vi "ReplaceInMatriceScaling.vi"(8 "Input Scaling":i32=4, 11 "Input Array":dbl[](array[numeric])) -> (0 "Output Array":dbl[][](array[numeric]))   [LabVIEW 2018]
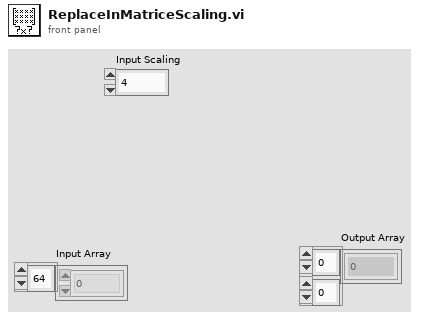
[diagram p1: front panel]
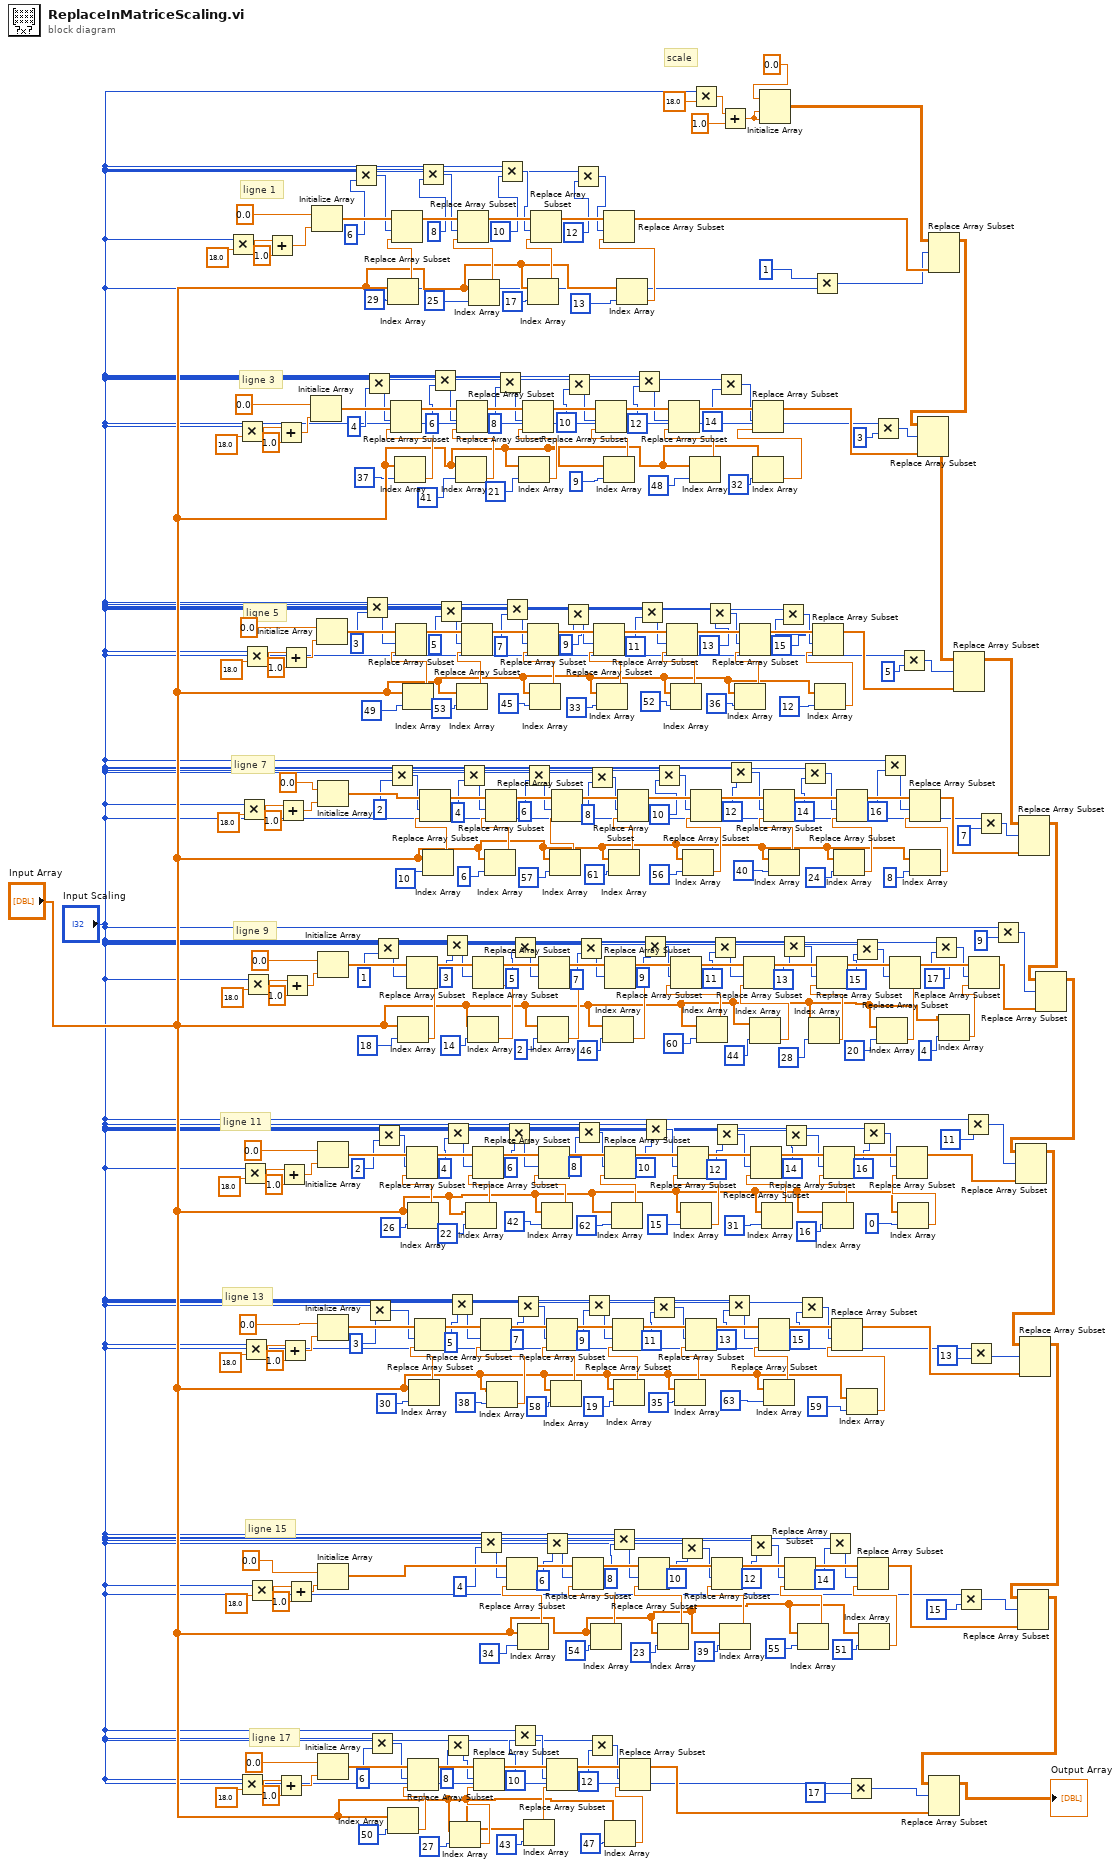
[diagram p0: block diagram]
diagram:
  # "scale"
  # "ligne 17"
  # "ligne 15"
  # "ligne 13"
  # "ligne 11"
  # "ligne 9"
  # "ligne 7"
  # "ligne 5"
  # "ligne 3"
  # "ligne 1"
  n1 = Multiply(x="Input Scaling", y=18.0) -> (x*y=w232:dbl)
  n2 = Multiply(x="Input Scaling", y=18.0) -> (x*y=w228:dbl)
  n3 = Multiply(x="Input Scaling", y=18.0) -> (x*y=w200:dbl)
  n4 = Multiply(x="Input Scaling", y=18.0) -> (x*y=w220:dbl)
  n5 = Multiply(x="Input Scaling", y=18.0) -> (x*y=w212:dbl)
  n6 = Multiply(x="Input Scaling", y=18.0) -> (x*y=w208:dbl)
  n7 = Multiply(x="Input Scaling", y=18.0) -> (x*y=w224:dbl)
  n8 = Multiply(x="Input Scaling", y=18.0) -> (x*y=w216:dbl)
  n9 = Multiply(x="Input Scaling", y=18.0) -> (x*y=w204:dbl)
  n10 = Add(x=w232, y=1.0) -> (x+y=w230:dbl)
  n11 = Add(x=w228, y=1.0) -> (x+y=w226:dbl)
  n12 = Add(x=w200, y=1.0) -> (x+y=w198:dbl)
  n13 = Add(x=w220, y=1.0) -> (x+y=w218:dbl)
  n14 = Add(x=w212, y=1.0) -> (x+y=w210:dbl)
  n15 = Add(x=w208, y=1.0) -> (x+y=w206:dbl)
  n16 = Add(x=w224, y=1.0) -> (x+y=w222:dbl)
  n17 = Add(x=w216, y=1.0) -> (x+y=w214:dbl)
  n18 = Add(x=w204, y=1.0) -> (x+y=w202:dbl)
  n19 = Initialize Array(0.0 ("element"), w226) -> (w372:dbl[])
  n20 = Initialize Array(0.0 ("element"), w230) -> (w382:dbl[])
  n21 = Initialize Array(0.0 ("element"), w222) -> (w365:dbl[])
  n22 = Initialize Array(0.0 ("element"), w218) -> (w356:dbl[])
  n23 = Initialize Array(0.0 ("element"), w214) -> (w347:dbl[])
  n24 = Initialize Array(0.0 ("element"), w210) -> (w338:dbl[])
  n25 = Initialize Array(0.0 ("element"), w206) -> (w330:dbl[])
  n26 = Initialize Array(0.0 ("element"), w202) -> (w322:dbl[])
  n27 = Initialize Array(0.0 ("element"), w198) -> (w320:dbl[])
  n28 = Multiply(x="Input Scaling", y=6 ("index")) -> (x*y=w195:i32)
  n29 = Multiply(x="Input Scaling", y=3 ("index")) -> (x*y=w176:i32)
  n30 = Multiply(x="Input Scaling", y=4 ("index")) -> (x*y=w187:i32)
  n31 = Multiply(x="Input Scaling", y=3 ("index")) -> (x*y=w112:i32)
  n32 = Multiply(x="Input Scaling", y=6 ("index")) -> (x*y=w86:i32)
  n33 = Multiply(x="Input Scaling", y=1 ("index")) -> (x*y=w146:i32)
  n34 = Multiply(x="Input Scaling", y=2 ("index")) -> (x*y=w128:i32)
  n35 = Multiply(x="Input Scaling", y=2 ("index")) -> (x*y=w162:i32)
  n36 = Index Array(array="Input Array", index=29) -> (element=w305:dbl)
  n37 = Index Array(array="Input Array", index=50) -> (element=w259:dbl)
  n38 = Replace Array Subset(array=w382, new element=w305, index=w195) -> (w381:dbl[])
  n39 = Index Array(array="Input Array", index=37) -> (element=w304:dbl)
  n40 = Replace Array Subset(array=w372, new element=w304, index=w187) -> (w373:dbl[])
  n41 = Index Array(array="Input Array", index=18) -> (element=w316:dbl)
  n42 = Index Array(array="Input Array", index=49) -> (element=w298:dbl)
  n43 = Replace Array Subset(array=w365, new element=w298, index=w176) -> (w366:dbl[])
  n44 = Replace Array Subset(array=w347, new element=w316, index=w146) -> (w346:dbl[])
  n45 = Index Array(array="Input Array", index=26) -> (element=w276:dbl)
  n46 = Replace Array Subset(array=w338, new element=w276, index=w128) -> (w339:dbl[])
  n47 = Replace Array Subset(array=w320, new element=w259, index=w86) -> (w319:dbl[])
  n48 = Index Array(array="Input Array", index=30) -> (element=w275:dbl)
  n49 = Replace Array Subset(array=w330, new element=w275, index=w112) -> (w331:dbl[])
  n50 = Multiply(x="Input Scaling", y=8 ("index")) -> (x*y=w190:i32)
  n51 = Index Array(array="Input Array", index=10) -> (element=w291:dbl)
  n52 = Replace Array Subset(array=w356, new element=w291, index=w162) -> (w357:dbl[])
  n53 = Multiply(x="Input Scaling", y=6 ("index")) -> (x*y=w185:i32)
  n54 = Multiply(x="Input Scaling", y=5 ("index")) -> (x*y=w174:i32)
  n55 = Multiply(x="Input Scaling", y=3 ("index")) -> (x*y=w144:i32)
  n56 = Multiply(x="Input Scaling", y=4 ("index")) -> (x*y=w126:i32)
  n57 = Multiply(x="Input Scaling", y=8 ("index")) -> (x*y=w84:i32)
  n58 = Multiply(x="Input Scaling", y=5 ("index")) -> (x*y=w110:i32)
  n59 = Index Array(array="Input Array", index=27) -> (element=w260:dbl)
  n60 = Index Array(array="Input Array", index=41) -> (element=w303:dbl)
  n61 = Replace Array Subset(array=w373, new element=w303, index=w185) -> (w377:dbl[])
  n62 = Index Array(array="Input Array", index=53) -> (element=w297:dbl)
  n63 = Multiply(x="Input Scaling", y=4 ("index")) -> (x*y=w160:i32)
  n64 = Replace Array Subset(array=w366, new element=w297, index=w174) -> (w370:dbl[])
  n65 = Index Array(array="Input Array", index=22) -> (element=w277:dbl)
  n66 = Index Array(array="Input Array", index=14) -> (element=w315:dbl)
  n67 = Index Array(array="Input Array", index=25) -> (element=w306:dbl)
  n68 = Replace Array Subset(array=w381, new element=w306, index=w190) -> (w380:dbl[])
  n69 = Replace Array Subset(array=w346, new element=w315, index=w144) -> (w349:dbl[])
  n70 = Replace Array Subset(array=w339, new element=w277, index=w126) -> (w340:dbl[])
  n71 = Replace Array Subset(array=w319, new element=w260, index=w84) -> (w318:dbl[])
  n72 = Multiply(x="Input Scaling", y=4 ("index")) -> (x*y=w98:i32)
  n73 = Index Array(array="Input Array", index=6) -> (element=w290:dbl)
  n74 = Replace Array Subset(array=w357, new element=w290, index=w160) -> (w358:dbl[])
  n75 = Index Array(array="Input Array", index=38) -> (element=w274:dbl)
  n76 = Replace Array Subset(array=w331, new element=w274, index=w110) -> (w335:dbl[])
  n77 = Multiply(x="Input Scaling", y=8 ("index")) -> (x*y=w184:i32)
  n78 = Multiply(x="Input Scaling", y=10 ("index")) -> (x*y=w191:i32)
  n79 = Multiply(x="Input Scaling", y=7 ("index")) -> (x*y=w172:i32)
  n80 = Multiply(x="Input Scaling", y=6 ("index")) -> (x*y=w124:i32)
  n81 = Multiply(x="Input Scaling", y=5 ("index")) -> (x*y=w142:i32)
  n82 = Multiply(x="Input Scaling", y=10 ("index")) -> (x*y=w82:i32)
  n83 = Multiply(x="Input Scaling", y=7 ("index")) -> (x*y=w108:i32)
  n84 = Index Array(array="Input Array", index=34) -> (element=w263:dbl)
  n85 = Replace Array Subset(array=w322, new element=w263, index=w98) -> (w323:dbl[])
  n86 = Index Array(array="Input Array", index=21) -> (element=w299:dbl)
  n87 = Replace Array Subset(array=w377, new element=w299, index=w184) -> (w376:dbl[])
  n88 = Multiply(x="Input Scaling", y=6 ("index")) -> (x*y=w157:i32)
  n89 = Index Array(array="Input Array", index=43) -> (element=w261:dbl)
  n90 = Index Array(array="Input Array", index=17) -> (element=w307:dbl)
  n91 = Index Array(array="Input Array", index=45) -> (element=w296:dbl)
  n92 = Replace Array Subset(array=w370, new element=w296, index=w172) -> (w369:dbl[])
  n93 = Replace Array Subset(array=w380, new element=w307, index=w191) -> (w379:dbl[])
  n94 = Index Array(array="Input Array", index=2) -> (element=w314:dbl)
  n95 = Replace Array Subset(array=w349, new element=w314, index=w142) -> (w353:dbl[])
  n96 = Index Array(array="Input Array", index=42) -> (element=w278:dbl)
  n97 = Replace Array Subset(array=w340, new element=w278, index=w124) -> (w344:dbl[])
  n98 = Multiply(x="Input Scaling", y=6 ("index")) -> (x*y=w96:i32)
  n99 = Replace Array Subset(array=w318, new element=w261, index=w82) -> (w317:dbl[])
  n100 = Index Array(array="Input Array", index=57) -> (element=w289:dbl)
  n101 = Index Array(array="Input Array", index=58) -> (element=w273:dbl)
  n102 = Replace Array Subset(array=w335, new element=w273, index=w108) -> (w334:dbl[])
  n103 = Replace Array Subset(array=w358, new element=w289, index=w157) -> (w362:dbl[])
  n104 = Multiply(x="Input Scaling", y=9 ("index")) -> (x*y=w170:i32)
  n105 = Multiply(x="Input Scaling", y=10 ("index")) -> (x*y=w182:i32)
  n106 = Multiply(x="Input Scaling", y=12 ("index")) -> (x*y=w194:i32)
  n107 = Multiply(x="Input Scaling", y=8 ("index")) -> (x*y=w122:i32)
  n108 = Multiply(x="Input Scaling", y=7 ("index")) -> (x*y=w140:i32)
  n109 = Multiply(x="Input Scaling", y=9 ("index")) -> (x*y=w106:i32)
  n110 = Multiply(x="Input Scaling", y=8 ("index")) -> (x*y=w156:i32)
  n111 = Multiply(x="Input Scaling", y=12 ("index")) -> (x*y=w80:i32)
  n112 = Index Array(array="Input Array", index=54) -> (element=w264:dbl)
  n113 = Replace Array Subset(array=w323, new element=w264, index=w96) -> (w327:dbl[])
  n114 = Index Array(array="Input Array", index=33) -> (element=w295:dbl)
  n115 = Replace Array Subset(array=w369, new element=w295, index=w170) -> (w368:dbl[])
  n116 = Index Array(array="Input Array", index=46) -> (element=w313:dbl)
  n117 = Index Array(array="Input Array", index=9) -> (element=w300:dbl)
  n118 = Replace Array Subset(array=w376, new element=w300, index=w182) -> (w375:dbl[])
  n119 = Replace Array Subset(array=w353, new element=w313, index=w140) -> (w352:dbl[])
  n120 = Index Array(array="Input Array", index=47) -> (element=w262:dbl)
  n121 = Index Array(array="Input Array", index=61) -> (element=w288:dbl)
  n122 = Multiply(x="Input Scaling", y=8 ("index")) -> (x*y=w94:i32)
  n123 = Index Array(array="Input Array", index=62) -> (element=w279:dbl)
  n124 = Replace Array Subset(array=w344, new element=w279, index=w122) -> (w343:dbl[])
  n125 = Index Array(array="Input Array", index=19) -> (element=w272:dbl)
  n126 = Replace Array Subset(array=w334, new element=w272, index=w106) -> (w333:dbl[])
  n127 = Index Array(array="Input Array", index=13) -> (element=w308:dbl)
  n128 = Replace Array Subset(array=w379, new element=w308, index=w194) -> (w257:dbl[])
  n129 = Replace Array Subset(array=w362, new element=w288, index=w156) -> (w361:dbl[])
  n130 = Replace Array Subset(array=w317, new element=w262, index=w80) -> (w242:dbl[])
  n131 = Multiply(x="Input Scaling", y=12 ("index")) -> (x*y=w180:i32)
  n132 = Multiply(x="Input Scaling", y=11 ("index")) -> (x*y=w168:i32)
  n133 = Multiply(x="Input Scaling", y=9 ("index")) -> (x*y=w138:i32)
  n134 = Multiply(x="Input Scaling", y=10 ("index")) -> (x*y=w120:i32)
  n135 = Multiply(x="Input Scaling", y=11 ("index")) -> (x*y=w104:i32)
  n136 = Multiply(x="Input Scaling", y=10 ("index")) -> (x*y=w154:i32)
  n137 = Index Array(array="Input Array", index=23) -> (element=w265:dbl)
  n138 = Replace Array Subset(array=w327, new element=w265, index=w94) -> (w326:dbl[])
  n139 = Index Array(array="Input Array", index=52) -> (element=w294:dbl)
  n140 = Replace Array Subset(array=w368, new element=w294, index=w168) -> (w367:dbl[])
  n141 = Index Array(array="Input Array", index=35) -> (element=w271:dbl)
  n142 = Multiply(x="Input Scaling", y=10 ("index")) -> (x*y=w92:i32)
  n143 = Index Array(array="Input Array", index=15) -> (element=w280:dbl)
  n144 = Replace Array Subset(array=w343, new element=w280, index=w120) -> (w342:dbl[])
  n145 = Index Array(array="Input Array", index=56) -> (element=w287:dbl)
  n146 = Replace Array Subset(array=w333, new element=w271, index=w104) -> (w332:dbl[])
  n147 = Index Array(array="Input Array", index=48) -> (element=w301:dbl)
  n148 = Replace Array Subset(array=w375, new element=w301, index=w180) -> (w374:dbl[])
  n149 = Multiply(x="Input Scaling", y=18.0) -> (x*y=w235:dbl)
  n150 = Replace Array Subset(array=w361, new element=w287, index=w154) -> (w360:dbl[])
  n151 = Index Array(array="Input Array", index=60) -> (element=w312:dbl)
  n152 = Replace Array Subset(array=w352, new element=w312, index=w138) -> (w351:dbl[])
  n153 = Multiply(x="Input Scaling", y=13 ("index")) -> (x*y=w166:i32)
  n154 = Multiply(x="Input Scaling", y=11 ("index")) -> (x*y=w136:i32)
  n155 = Multiply(x="Input Scaling", y=12 ("index")) -> (x*y=w118:i32)
  n156 = Multiply(x="Input Scaling", y=14 ("index")) -> (x*y=w178:i32)
  n157 = Add(x=w235, y=1.0) -> (x+y=w236:dbl)
  n158 = Index Array(array="Input Array", index=39) -> (element=w266:dbl)
  n159 = Replace Array Subset(array=w326, new element=w266, index=w92) -> (w325:dbl[])
  n160 = Multiply(x="Input Scaling", y=13 ("index")) -> (x*y=w102:i32)
  n161 = Multiply(x="Input Scaling", y=12 ("index")) -> (x*y=w152:i32)
  n162 = Index Array(array="Input Array", index=36) -> (element=w293:dbl)
  n163 = Replace Array Subset(array=w367, new element=w293, index=w166) -> (w364:dbl[])
  n164 = Multiply(x="Input Scaling", y=12 ("index")) -> (x*y=w90:i32)
  n165 = Index Array(array="Input Array", index=44) -> (element=w311:dbl)
  n166 = Replace Array Subset(array=w351, new element=w311, index=w136) -> (w350:dbl[])
  n167 = Index Array(array="Input Array", index=32) -> (element=w302:dbl)
  n168 = Replace Array Subset(array=w374, new element=w302, index=w178) -> (w248:dbl[])
  n169 = Initialize Array(0.0, w236, w236) -> (w258:dbl[][])
  n170 = Index Array(array="Input Array", index=31) -> (element=w281:dbl)
  n171 = Replace Array Subset(array=w342, new element=w281, index=w118) -> (w341:dbl[])
  n172 = Index Array(array="Input Array", index=63) -> (element=w270:dbl)
  n173 = Replace Array Subset(array=w332, new element=w270, index=w102) -> (w329:dbl[])
  n174 = Index Array(array="Input Array", index=40) -> (element=w286:dbl)
  n175 = Replace Array Subset(array=w360, new element=w286, index=w152) -> (w359:dbl[])
  n176 = Multiply(x="Input Scaling", y=15 ("index")) -> (x*y=w164:i32)
  n177 = Multiply(x="Input Scaling", y=13 ("index")) -> (x*y=w134:i32)
  n178 = Multiply(x="Input Scaling", y=14 ("index")) -> (x*y=w116:i32)
  n179 = Multiply(x="Input Scaling", y=15 ("index")) -> (x*y=w100:i32)
  n180 = Index Array(array="Input Array", index=55) -> (element=w267:dbl)
  n181 = Replace Array Subset(array=w325, new element=w267, index=w90) -> (w324:dbl[])
  n182 = Multiply(x="Input Scaling", y=14 ("index")) -> (x*y=w150:i32)
  n183 = Index Array(array="Input Array", index=28) -> (element=w310:dbl)
  n184 = Multiply(x=1 ("index (row)"), y="Input Scaling") -> (x*y=w77:i32)
  n185 = Index Array(array="Input Array", index=12) -> (element=w292:dbl)
  n186 = Replace Array Subset(array=w364, new element=w292, index=w164) -> (w247:dbl[])
  n187 = Replace Array Subset(array=w350, new element=w310, index=w134) -> (w348:dbl[])
  n188 = Index Array(array="Input Array", index=16) -> (element=w282:dbl)
  n189 = Replace Array Subset(array=w341, new element=w282, index=w116) -> (w337:dbl[])
  n190 = Multiply(x="Input Scaling", y=14 ("index")) -> (x*y=w88:i32)
  n191 = Index Array(array="Input Array", index=24) -> (element=w285:dbl)
  n192 = Replace Array Subset(array=w359, new element=w285, index=w150) -> (w355:dbl[])
  n193 = Multiply(x="Input Scaling", y=17 ("index (row)")) -> (x*y=w62:i32)
  n194 = Index Array(array="Input Array", index=59) -> (element=w269:dbl)
  n195 = Replace Array Subset(array=w329, new element=w269, index=w100) -> (w244:dbl[])
  n196 = Multiply(x="Input Scaling", y=15 ("index")) -> (x*y=w132:i32)
  n197 = Multiply(x="Input Scaling", y=16 ("index")) -> (x*y=w114:i32)
  n198 = Index Array(array="Input Array", index=51) -> (element=w268:dbl)
  n199 = Replace Array Subset(array=w324, new element=w268, index=w88) -> (w243:dbl[])
  n200 = Multiply(x="Input Scaling", y=3 ("index (row)")) -> (x*y=w76:i32)
  n201 = Index Array(array="Input Array", index=20) -> (element=w309:dbl)
  n202 = Multiply(x="Input Scaling", y=16 ("index")) -> (x*y=w148:i32)
  n203 = Replace Array Subset(array=w348, new element=w309, index=w132) -> (w240:dbl[])
  n204 = Index Array(array="Input Array", index=0) -> (element=w283:dbl)
  n205 = Replace Array Subset(array=w337, new element=w283, index=w114) -> (w245:dbl[])
  n206 = Multiply(x="Input Scaling", y=5 ("index (row)")) -> (x*y=w73:i32)
  n207 = Index Array(array="Input Array", index=8) -> (element=w284:dbl)
  n208 = Replace Array Subset(array=w355, new element=w284, index=w148) -> (w246:dbl[])
  n209 = Replace Array Subset(array=w258, new element=w257, index (row)=w77) -> (w256:dbl[][])  [unwired: 1 in]
  n210 = Replace Array Subset(array=w256, new element=w248, index (row)=w76) -> (w255:dbl[][])  [unwired: 1 in]
  n211 = Multiply(x="Input Scaling", y=17 ("index")) -> (x*y=w130:i32)
  n212 = Index Array(array="Input Array", index=4) -> (element=w238:dbl)
  n213 = Replace Array Subset(array=w255, new element=w247, index (row)=w73) -> (w254:dbl[][])  [unwired: 1 in]
  n214 = Multiply(x="Input Scaling", y=15 ("index (row)")) -> (x*y=w63:i32)
  n215 = Multiply(x="Input Scaling", y=11 ("index (row)")) -> (x*y=w67:i32)
  n216 = Multiply(x="Input Scaling", y=13 ("index (row)")) -> (x*y=w66:i32)
  n217 = Replace Array Subset(array=w240, new element=w238, index=w130) -> (w239:dbl[])
  n218 = Multiply(x="Input Scaling", y=7 ("index (row)")) -> (x*y=w71:i32)
  n219 = Multiply(x="Input Scaling", y=9 ("index (row)")) -> (x*y=w70:i32)
  n220 = Replace Array Subset(array=w254, new element=w246, index (row)=w71) -> (w253:dbl[][])  [unwired: 1 in]
  n221 = Replace Array Subset(array=w253, new element=w239, index (row)=w70) -> (w252:dbl[][])  [unwired: 1 in]
  n222 = Replace Array Subset(array=w252, new element=w245, index (row)=w67) -> (w251:dbl[][])  [unwired: 1 in]
  n223 = Replace Array Subset(array=w251, new element=w244, index (row)=w66) -> (w250:dbl[][])  [unwired: 1 in]
  n224 = Replace Array Subset(array=w250, new element=w243, index (row)=w63) -> (w249:dbl[][])  [unwired: 1 in]
  n225 = Replace Array Subset(array=w249, new element=w242, index (row)=w62) -> (→"Output Array":dbl[][])  [unwired: 1 in]
